vi "ex_1.vi"() -> ()   [LabVIEW 2020]
panel:
  in  "dx":dbl
  out "Waveform Chart":dbl(graph)
  out "Waveform Graph 2":cluster{"x":dbl, "dx":dbl, dbl[]}(graph)
  in  "dx 2":dbl
  in  "stop":bool
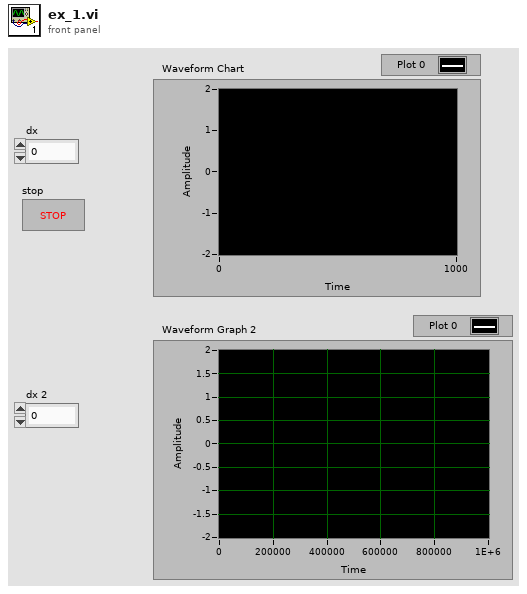
[diagram p1: front panel]
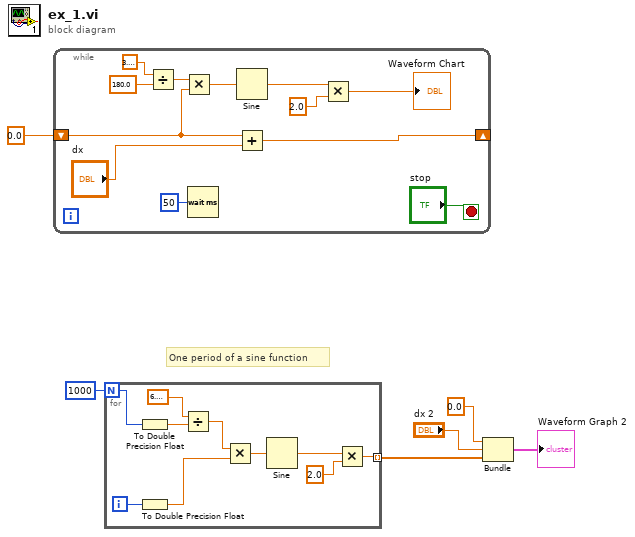
[diagram p0: block diagram]
diagram:
  # "One period of a sine function"
  n1 = while {
    shift-right: [w9] -> _
    shift-left: 0.0 -> [w8]
    stop <- "stop" stop-if-true
    n2 = Divide(x=3.141592653589793, y=180.0) -> (x/y=w10:dbl)
    n3 = Multiply(x=w10, y=w8) -> (x*y=w14:dbl)
    n4 = Wait (ms)(milliseconds to wait=u32 50) -> ()  [unwired: 1 out]
    n5 = Sine(x=w14) -> (sin(x)=w18:dbl)
    n6 = Add(x=w8, y="dx") -> (x+y=w9:dbl)
    n7 = Multiply(x=w18, y=2.0) -> (x*y=→"Waveform Chart":dbl)
  }
  n8 = for {
    N: 1000 -> [w28]
    tunnel: [w20] -> w2 mode=indexing
    i -> [w26]
    n9 = To Double Precision Float(number=w28) -> (double precision float=w23:dbl)
    n10 = To Double Precision Float(number=w26) -> (double precision float=w25:dbl)
    n11 = Divide(x=6.283185307179586, y=w23) -> (x/y=w27:dbl)
    n12 = Multiply(x=w27, y=w25) -> (x*y=w24:dbl)
    n13 = Sine(x=w24) -> (sin(x)=w21:dbl)
    n14 = Multiply(x=w21, y=2.0) -> (x*y=w20:dbl)
  }
  n15 = Bundle("x"=0.0, "dx 2"="dx 2", w2) -> (→"Waveform Graph 2":cluster{"x":dbl, "dx 2":dbl, dbl[]})  [unwired: 1 in]
